vi "GPIO.vi"(11 "AnalogIn in":refnum<class "AI.lvclass">) -> (2 "GPIO":refnum<class "GPIO.lvclass">)   [LabVIEW 2024, in "CTI.lvlib" / "AI.lvclass"]
uses:
  AI.lvclass
  GPIO/GPIO.lvclass
  AI.lvclass/AI.ctl
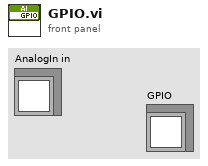
[diagram p1: front panel]
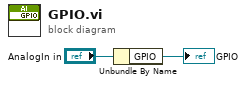
[diagram p0: block diagram]
diagram:
  n1 = Unbundle By Name("AnalogIn in") -> ("GPIO"=→"GPIO":refnum<class "GPIO.lvclass">)
